vi "ziModSetValue.vi"   [LabVIEW 2009, in "Zurich Instruments LabOne.lvlib"]
doc: "This polymorphic vi sets values to <b>module</b> nodes specified by <b>Path</b> to <b>Value</b>."
uses:
  <instrlib>/Zurich Instruments LabOne/Zurich Instruments LabOne.lvlib
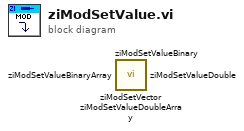
[diagram p0: block diagram]
diagram:
  n1 = call <instrlib>:"ziModSetVector.vi"() -> ()  [unwired: 10 in, 2 out]
  n2 = call <instrlib>:"ziModSetValueBinary.vi"() -> ()  [unwired: 10 in, 2 out]
  n3 = call <instrlib>:"ziModSetValueBinaryArray.vi"() -> ()  [unwired: 10 in, 2 out]
  n4 = call <instrlib>:"ziModSetValueDouble.vi"() -> ()  [unwired: 10 in, 2 out]
  n5 = call <instrlib>:"ziModSetValueDoubleArray.vi"() -> ()  [unwired: 10 in, 2 out]
